vi "led blink.vi"() -> ()   [LabVIEW 2020]
panel:
  out "Array":bool[][](array[boolean])
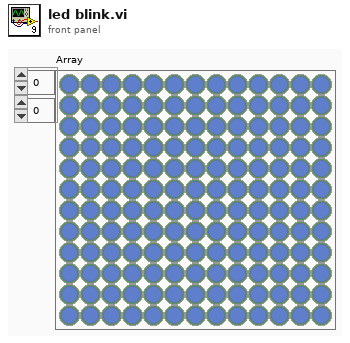
[diagram p1: front panel]
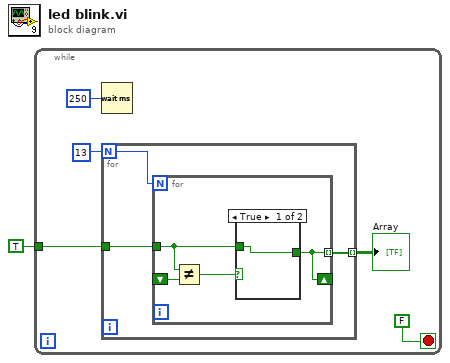
[diagram p0: block diagram]
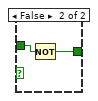
[diagram p2: hidden frame]
diagram:
  n1 = while {
    tunnel: TRUE -> [w2]
    stop <- FALSE stop-if-true
    n2 = Wait (ms)(milliseconds to wait=u32 250) -> ()  [unwired: 1 out]
    n3 = for {
      N: 13 -> [w7]
      tunnel: [w9] -> w3 mode=indexing
      tunnel: w2 -> [w8]
      n4 = for {
        N: w7 -> [_]
        tunnel: [w10] -> w9 mode=indexing
        tunnel: w8 -> [w12]
        shift-right: [w10] -> _
        shift-left: _ -> [w11]
        n5 = Not Equal?(x=w12, y=w11) -> (x != y?=w13:bool)
        n6 = case shown="True" w13 {
          tunnel: [w14 w16] -> w10
          tunnel: w12 -> [w14 w15]
          frame True {
          }
          frame False {
            n7 = Not(x=w15) -> (.not. x?=w16:bool)
          }
        }
      }
    }
    "Array" <- w3
  }
